vi "GetError.vi"(0 "Fehler (Eingang, kein Fehler)":errorcluster, 5 "instanceHandle":u32, 7 "DLL-Path":path, 9 "maxLen":u32) -> (4 "Fehler (Ausgang)":errorcluster, 6 "instanceHandle":u32, 8 "DLL-Path":path, 10 "ERR_CODE":i32, 15 "errText":string)   [LabVIEW 2015, in "MEDAQLib.lvlib"]
doc: "ERR_CODE GetError (DWORD instanceHandle, LPTSTR errText, DWORD maxLen);\n\nGet the last error in driver.\nThis function can be used after an error return from function OpenSensor,\nCloseSensor, SensorCommand, DataAvail, TransferData and Poll.\nFor all functions above and error code ERR_INSTANCE_NOT_EXIST this func-\ntion does not return an error text.\nFor function DataAvail and error code ERR_WRONG_PARAMETER this func-\ntion does not return an error text."
uses:
  MEDAQLib.lvlib
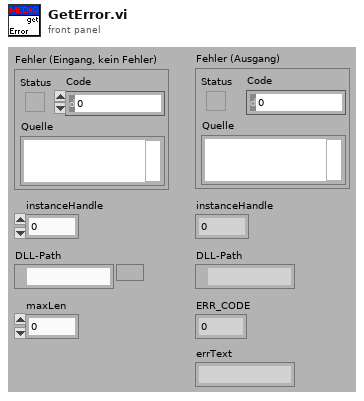
[diagram p1: front panel]
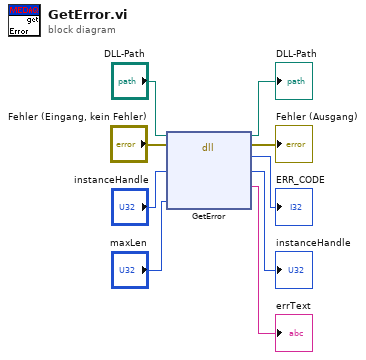
[diagram p0: block diagram]
diagram:
  n1 = dll-call lib="C:/Programme/National Instruments 8.6/LabVIEW 8.6/instr.lib/MEDAQLib/Release/MEDAQLib.dll" fn="GetError"(path in="DLL-Path", error in="Fehler (Eingang, kein Fehler)", "instanceHandle"="instanceHandle", "maxLen"="maxLen") -> (path out=→"DLL-Path":path, error out=→"Fehler (Ausgang)":errorcluster, "Rückgabetyp"=→"ERR_CODE":i32, "instanceHandle"=→"instanceHandle":u32, "errText"=→"errText":string)  [unwired: 2 in, 1 out]
